vi "WalkOnSuite.vi"(6 "Stop on 1st fail":bool, 7 "Banana":refnum<class "Banana.lvclass">, 8 "error in (no error)":errorcluster, 10 "Properties.Suite":refnum<class "Properties.Suite.lvclass">) -> (0 "error out":errorcluster, 2 "Properties.Suite out":refnum<class "Properties.Suite.lvclass">)   [LabVIEW 2021, in "Bananas.lvlib" / "Platano.lvclass"]
uses:
  Platano/Platano.lvclass
  BananaPeel/BananaPeel.lvclass
  Banana.lvclass
  <vilib>/addons/_JKI Toolkits/Caraya/classes/Properties.Suite/Properties.Suite.lvclass
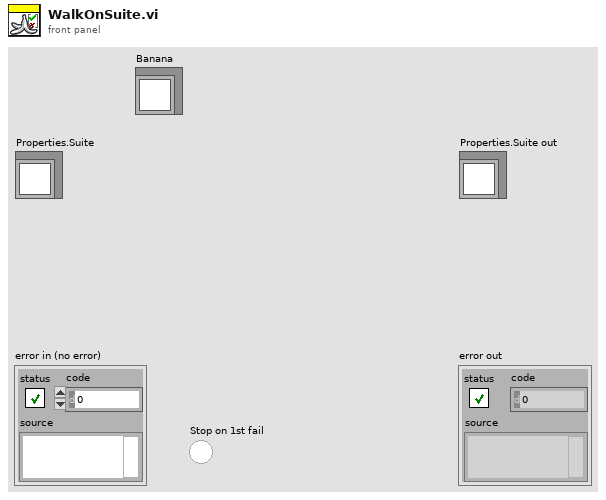
[diagram p1: front panel]
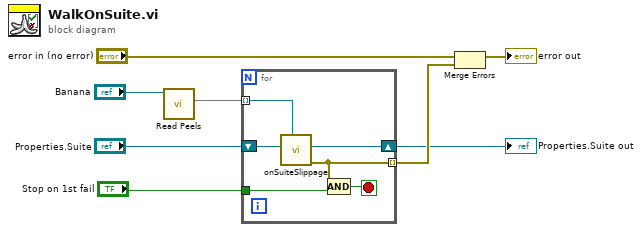
[diagram p0: block diagram]
diagram:
  n1 = call "Read Peels.vi"("Banana in"="Banana") -> ("Peels"=w1:set{refnum<class "BananaPeel.lvclass">})  [unwired: 8 in, 2 out]
  n2 = for {
    tunnel: [w9] -> w8 mode=indexing
    shift-right: [w10] -> w5
    shift-left: "Properties.Suite" -> [w11]
    tunnel: w1 -> [w12] mode=indexing
    tunnel: "Stop on 1st fail" -> [w14]
    stop <- w13 stop-if-true
    n3 = call-dynamic "onSuiteSlippage.vi"("BananaPeel in"=w12, "Properties.Suite"=w11) -> ("error out"=w9:errorcluster, "Properties.Suite out"=w10:refnum<class "Properties.Suite.lvclass">)  [unwired: 8 in]
    n4 = Compound Arithmetic op=AND(w9, w14) -> (w13:bool)
  }
  "Properties.Suite out" <- w5
  n5 = Merge Errors("error in (no error)", w8) -> (→"error out":errorcluster)
